vi "ROI2Mask.vi"() -> ()   [LabVIEW 2016]
doc: "This example shows how to compute the histogram of an image or a region in the image. This example also shows how to set up and use the display tools to select and work on different regions in the image interactively."
uses:
  <vilib>/vision/NI_Vision_Development_Module.lvlib
panel:
  out "Mean":sgl format="%#.2f"
  out "Standard Deviation":sgl format="%#.2f"
  out "Image":T1(plugin-control)
  out "Histogram":T2(graph)
  in  "Stop":bool
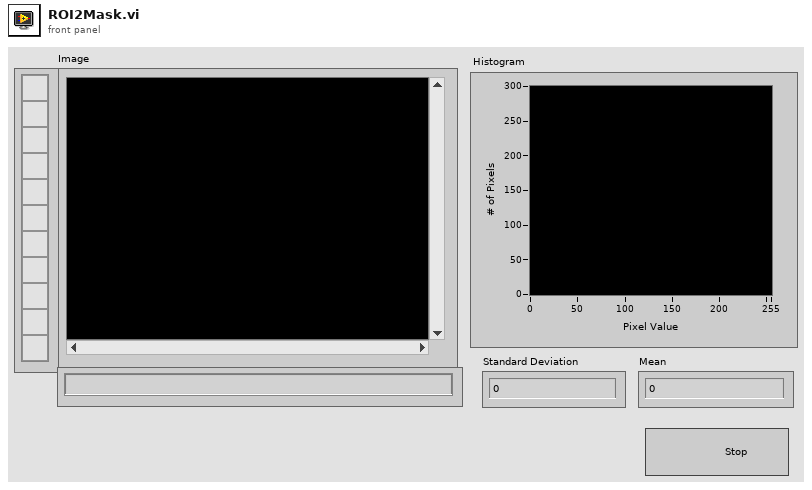
[diagram p1: front panel]
types:
  T1 = typedef "IMAQ Image.ctl" = refnum<image>
  T2 = cluster{"Starting Value":sgl, "Incremental Value":sgl, "Histogram":u32[]}
  T3 = typedef "IMAQ Rectangle" = cluster{"Left":i32, "Top":i32, "Right":i32, "Bottom":i32, "Rotation":dbl}
  T4 = typedef "ROI Descriptor" = cluster{"Global Rectangle":i32[], "Contours":cluster{"ID":enum32{"External", "Internal"}, "Type":u32, "Coordinates":i32[]}[]}
  T5 = cluster{"Global Rectangle":i32[], "Contours":cluster{"Contour Type":u32, "ROI Type":u32, "Points":i32[]}[]}
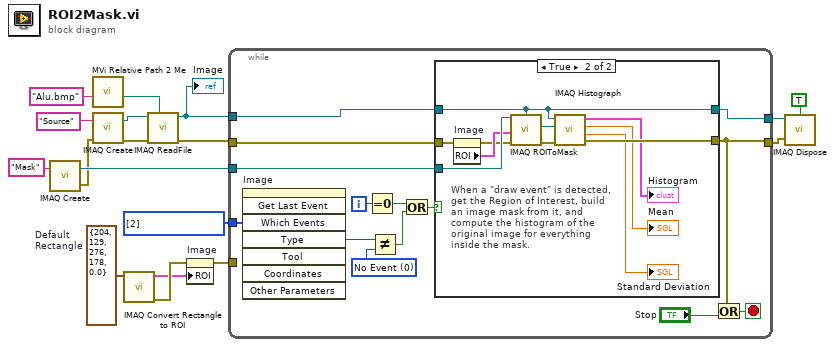
[diagram p0: block diagram]
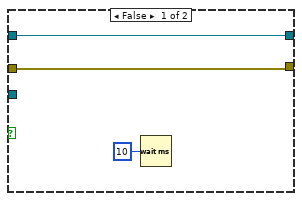
[diagram p2: hidden frame]
diagram:
  w8 = T3 {"Left"=204, "Top"=129, "Right"=276, "Bottom"=178, "Rotation"=0.0}  # Default  Rectangle
  w11 = i32[] [2] items=["No  event", "Click event", "Draw event", "Move event", "Size event", "Scroll event", "Activate event", "Close event", "Double click event"] ("Events list (all)")
  n1 = call "IMAQ Create"("Image Name"="Mask") -> ("New Image"=w13:T1, "error out"=w6:errorcluster)  [unwired: 4 in]
  n2 = call "MVi Relative Path 2 Me.vi"("Relative Path"="Alu.bmp") -> ("Appended Dir"=w2:path)  [unwired: 5 in, 1 out]
  n3 = call "IMAQ Create"("Image Name"="Source", "error in (no error)"=w6) -> ("New Image"=w18:T1, "error out"=w17:errorcluster)  [unwired: 3 in]
  n4 = call "IMAQ Convert Rectangle to ROI"("Rectangle"=w8) -> ("error out"=w7:errorcluster, "ROI Descriptor"=w5:T4)  [unwired: 8 in]
  n5 = call "IMAQ ReadFile"("File Path"=w2, "error in (no error)"=w17, "Image"=w18) -> ("error out"=w15:errorcluster, "Image Out"=w9:T1)  [unwired: 4 in, 3 out]
  "Image" <- w9
  n6 = property on="Image" class="ImageControl"(error in=w7, "ROI"=w5) -> (error out=w4:errorcluster)  [unwired: 1 in, 1 out]
  n7 = while {
    tunnel: w9 -> [w27]
    tunnel: w15 -> [w28]
    tunnel: w13 -> [w29]
    tunnel: [w25] -> w12
    tunnel: [w31] -> w10
    tunnel: w11 -> [w26]
    tunnel: w4 -> [_]
    i -> [w23]
    stop <- w30 stop-if-true
    w20 = 0 items=["No Event"=0, "Click Event"=1, "Draw Event"=2, "Size Event"=4, "Scroll Event"=5, "Double Click Event"=8] ("Type")
    n8 = invoke on="Image" class="ImageControl" method="Get Last Event"("Which Events"=w26) -> ("Type"=w21:i32)  [unwired: 7 in, 7 out]
    n9 = Equal To 0?(x=w23) -> (x = 0?=w22:bool)
    n10 = Not Equal?(x=w21, y=w20) -> (x != y?=w19:bool)
    n11 = Or(x=w22, y=w19) -> (x .or. y?=w24:bool)
    n12 = case shown="True" w24 {
      tunnel: w27 -> [w34 w41]
      tunnel: w29 -> [_ w42]
      tunnel: [w33 w44] -> w25
      tunnel: [w34 w41] -> w31
      tunnel: w28 -> [w33 w40]
      frame False {
        n13 = Wait (ms)(milliseconds to wait=u32 10) -> ()  [unwired: 1 out]
      }
      frame True {
        # "When a \"draw event\" is detected, get the Region of Interest, build an image mask from it, and compute the histogram of the original image for everything inside the mask."
        n14 = property on="Image" class="ImageControl"(error in=w40) -> (error out=w38:errorcluster, "ROI"=w39:T5)  [unwired: 1 in, 1 out]
        n15 = call "IMAQ ROIToMask"("error in (no error)"=w38, "ROI Descriptor"=w39, "Image"=w42, "Image Model"=w41) -> ("error out"=w45:errorcluster, "Image Out"=w46:T1)  [unwired: 2 in, 1 out]
        n16 = call "IMAQ Histograph"("error in (no error)"=w45, "Image Mask"=w46, "Image"=w41) -> ("error out"=w44:errorcluster, "Standard  Deviation"=→"Standard Deviation":sgl, "Mean Value"=→"Mean":sgl, "Histogram Graph"=→"Histogram":T2)  [unwired: 5 in]
      }
    }
    n17 = Or(x=w25, y="Stop") -> (x .or. y?=w30:bool)
  }
  n18 = call "IMAQ Dispose"("All Images? (No)"=TRUE, "Image"=w10, "error in (no error)"=w12) -> ()  [unwired: 3 in, 1 out]
